vi "channel2Platform.vi"(9 "mazeDirection":string, 11 "DAQmx \nPhysical Channel":tag="Dev2/ai0:31") -> (3 "Platform number":i32)   [LabVIEW 2017]
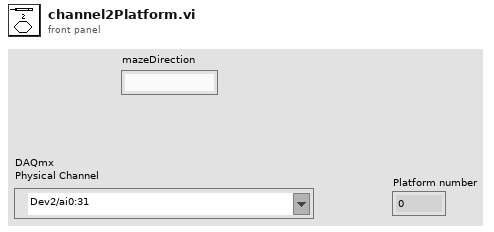
[diagram p1: front panel]
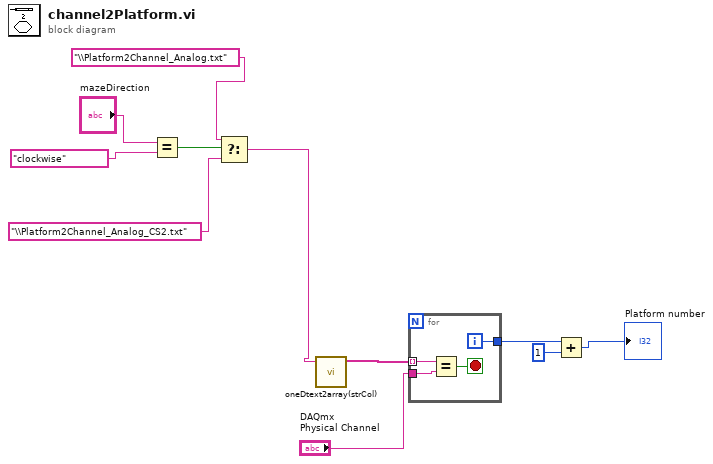
[diagram p0: block diagram]
diagram:
  n1 = Equal?(x="mazeDirection", y="clockwise") -> (x = y?=w4:bool)
  n2 = Select(t="\\Platform2Channel_Analog.txt" ("String"), s=w4, f="\\Platform2Channel_Analog_CS2.txt" ("String")) -> (s? t:f=w1:string)
  n3 = call "oneDtext2array(strCol).vi"("String"=w1) -> ("text"=w11:string[])  [unwired: 10 in]
  n4 = for {
    tunnel: w11 -> [w15] mode=indexing
    tunnel: "DAQmx \nPhysical Channel" -> [w14]
    tunnel: [w13] -> w9
    i -> [w13]
    stop <- w12 stop-if-true
    n5 = Equal?(x=w15, y=w14) -> (x = y?=w12:bool)
  }
  n6 = Add(x=w9, y=1) -> (x+y=→"Platform number":i32)
